vi "User Defined Errors.vi"(8 "error in (no error)":errorcluster, 9 "Parameter 2":string, 10 "Parameter 1":string, 11 "Error Code (0)":i32=-1) -> (0 "error out":errorcluster)   [LabVIEW 2024]
doc: "Returns the error by specifying the error code."
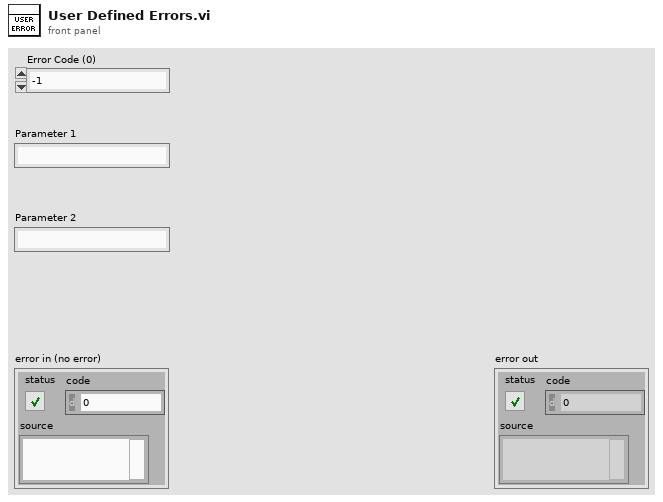
[diagram p1: front panel]
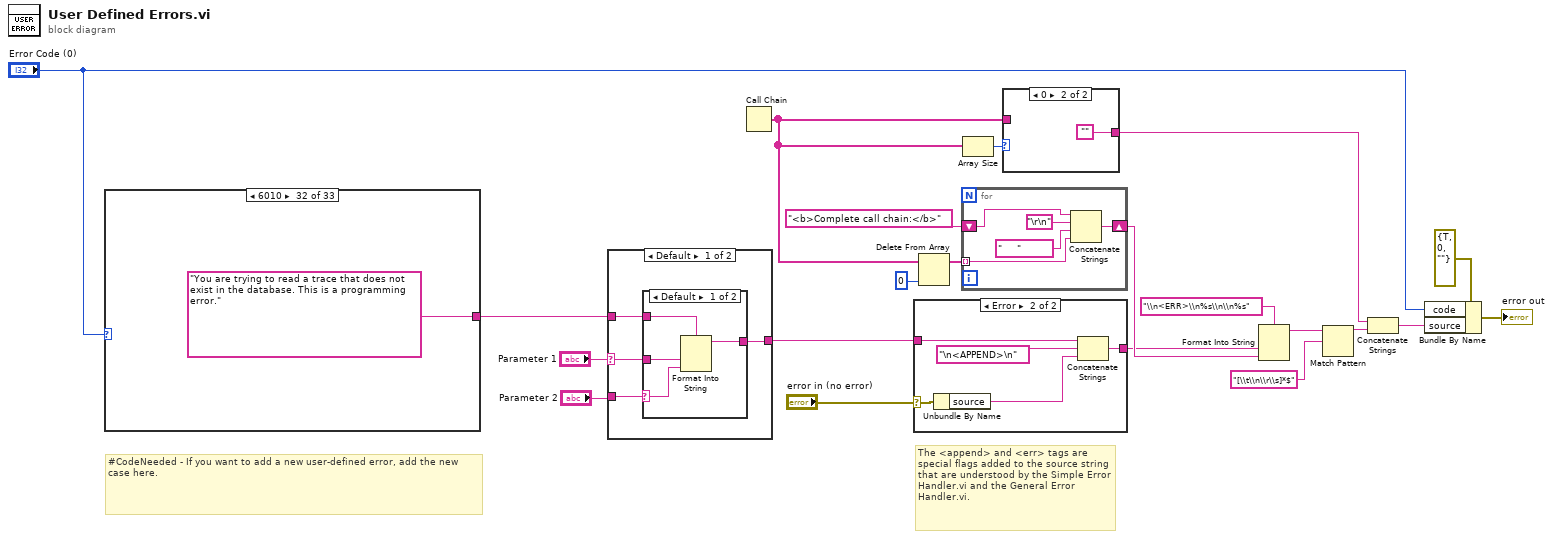
[diagram p0: block diagram]
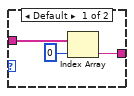
[diagram p2: hidden frame]
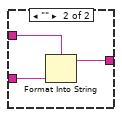
[diagram p4: hidden frame]
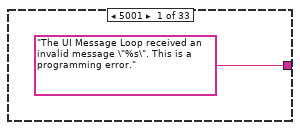
[diagram p6: hidden frame]
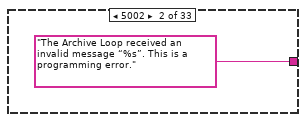
[diagram p7: hidden frame]
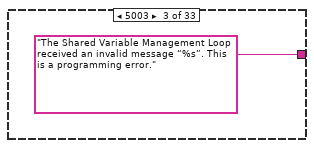
[diagram p8: hidden frame]
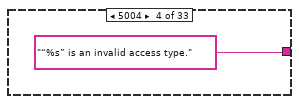
[diagram p9: hidden frame]
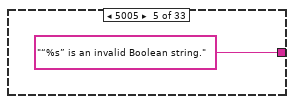
[diagram p10: hidden frame]
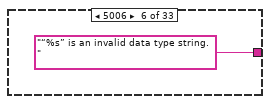
[diagram p11: hidden frame]
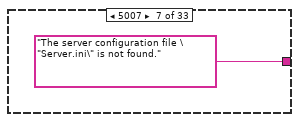
[diagram p12: hidden frame]
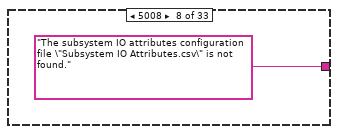
[diagram p13: hidden frame]
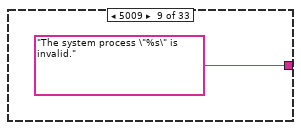
[diagram p14: hidden frame]
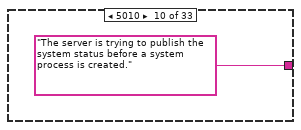
[diagram p15: hidden frame]
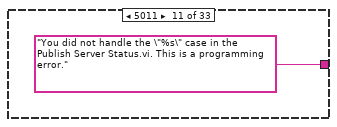
[diagram p16: hidden frame]
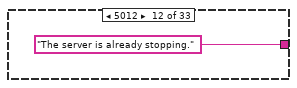
[diagram p17: hidden frame]
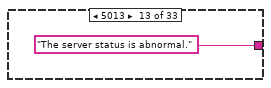
[diagram p18: hidden frame]
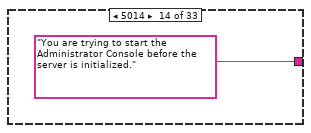
[diagram p19: hidden frame]
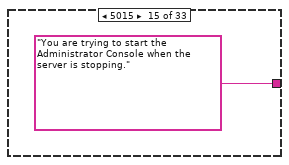
[diagram p20: hidden frame]
diagram:
  # "#CodeNeeded - If you want to add a new user-defined error, add the new case here."
  # "The <append> and <err> tags are special flags added to the source string that are understood by the Simple Error Handler.vi and the General Error Handler.vi."
  n1 = case shown="6010" "Error Code (0)" {
    selector: "Error Code (0)" -> [_ _ _ _ _ _ _ _ _ _ _ _ _ _ _ _ _ _ _ _ _ _ _ _ _ _ _ _ _ _ _ _ w55]
    tunnel: ["The UI Message Loop received an invalid message \"%s\". This is a programming error." ("Invalid Logging Message") "The Archive Loop received an invalid message “%s”. This is a programming error." ("Invalid Logging Message") "The Shared Variable Management Loop received an invalid message “%s”. This is a programming error." ("Unknown Message Error Text") "“%s” is an invalid access type." ("Invalid Logging Message") "“%s” is an invalid Boolean string." ("Invalid Logging Message") "“%s” is an invalid data type string. " ("Invalid Logging Message") "The server configuration file \"Server.ini\" is not found." ("Invalid Logging Message") "The subsystem IO attributes configuration file \"Subsystem IO Attributes.csv\" is not found." ("Invalid Logging Message") "The system process \"%s\" is invalid." ("Invalid Logging Message") "The server is trying to publish the system status before a system process is created." ("Invalid Logging Message") "You did not handle the \"%s\" case in the Publish Server Status.vi. This is a programming error." ("message") "The server is already stopping." ("message") "The server status is abnormal." ("error message (\"\")") "You are trying to start the Administrator Console before the server is initialized." ("message") "You are trying to start the Administrator Console when the server is stopping." ("message") "The shared variable management failed to initialize." ("Invalid Logging Message") "The system configuration update failed." ("Invalid Logging Message") "A timer error occurred." ("Invalid Logging Message") "The archival failed." ("message") "The Administrator Console received an invalid message \"%s\". This is a programming error." ("message") "The archival configuration update failed." ("message") "The archival initialization failed." ("message") "The Message Handling Loop in the Client Main.vi received an invalid message “%s”. This is a programming error." ("Invalid Logging Message") "The Message Handling Loop in the Detailed View.vi received an invalid message “%s”. This is a programming error." ("Invalid Logging Message") "You are trying to switch to another detailed subview  with the \"%s\" command. But you did not create a corresponding switching case in the Open Subview VI Reference.vi. This is a programming error." ("message") "The string \"%s\" already exists in the list." "The string \"%s\" is already removed from the list." "Failed to read the historical data." "The array size of the data exceeds the maximum value of the array size. This is a programming error." "The client configuration file \"Client.ini\" is not found." ("message") "You are trying to bind the control \"%s\" to an item. But you did not create a corresponding binding case in advance. This is a programming error." ("message") "You are trying to read a trace that does not exist in the database. This is a programming error." ("message") w54] -> w21
    frame 5001 {
    }
    frame 5002 {
    }
    frame 5003 {
    }
    frame 5004 {
    }
    frame 5005 {
    }
    frame 5006 {
    }
    frame 5007 {
    }
    frame 5008 {
    }
    frame 5009 {
    }
    frame 5010 {
    }
    frame 5011 {
    }
    frame 5012 {
    }
    frame 5013 {
    }
    frame 5014 {
    }
    frame 5015 {
    }
    frame 5016 {
    }
    frame 5017 {
    }
    frame 5018 {
    }
    frame 5019 {
    }
    frame 5020 {
    }
    frame 5021 {
    }
    frame 5022 {
    }
    frame 6001 {
    }
    frame 6002 {
    }
    frame 6003 {
    }
    frame 6004 {
    }
    frame 6005 {
    }
    frame 6006 {
    }
    frame 6007 {
    }
    frame 6008 {
    }
    frame 6009 {
    }
    frame 6010 {
    }
    frame Default {
      n2 = Format Into String(format string="The error code \"%d\" is not defined. " ("Unknown Message Error Text"), w55) -> (resulting string=w54:string)  [unwired: 2 in, 1 out]
    }
  }
  n3 = case shown="Default" "Parameter 1" {
    selector: "Parameter 1" -> [w58 _]
    tunnel: [w60 w68] -> w5
    tunnel: w21 -> [w59 w68]
    tunnel: "Parameter 2" -> [w57 _]
    frame Default {
      n4 = case shown="Default" w57 {
        selector: w57 -> [w61 _]
        tunnel: w58 -> [w64 w67]
        tunnel: [w63 w66] -> w60
        tunnel: w59 -> [w62 w65]
        frame Default {
          n5 = Format Into String(format string=w62, w64, w61) -> (resulting string=w63:string)  [unwired: 2 in, 1 out]
        }
        frame "" {
          n6 = Format Into String(format string=w65, w67) -> (resulting string=w66:string)  [unwired: 2 in, 1 out]
        }
      }
    }
    frame "" {
    }
  }
  n7 = Call Chain() -> (call chain=w2:string[])
  n8 = case shown="Error" "error in (no error)" {
    selector: "error in (no error)" -> [_ w73]
    tunnel: [w69 w74] -> w4
    tunnel: w5 -> [w69 w70]
    frame No Error {
    }
    frame Error {
      n9 = Unbundle By Name(w73) -> ("source"=w72:string)
      n10 = Concatenate Strings(w70, "\n<APPEND>\n", w72) -> (w74:string)
    }
  }
  n11 = Delete From Array(array=w2, index=0) -> (array with subset deleted=w13:string[])  [unwired: 1 in, 1 out]
  n12 = for {
    tunnel: w13 -> [w76] mode=indexing
    shift-right: [w79] -> w7
    shift-left: "<b>Complete call chain:</b>" ("call chain header") -> [w77]
    n13 = Concatenate Strings(w77, "\r\n", "     ", w76) -> (w79:string)
  }
  n14 = Array Size(array=w2) -> (size(s)=w3:i32)
  n15 = case shown="0" w3 {
    tunnel: w2 -> [w81 _]
    tunnel: [w80 ""] -> w1
    frame Default {
      n16 = Index Array(array=w81, index=0) -> (element=w80:string)
    }
    frame 0 {
    }
  }
  n17 = Format Into String(format string="\\n<ERR>\\n%s\\n\\n%s", w4, w7) -> (resulting string=w15:string)  [unwired: 2 in, 1 out]
  n18 = Match Pattern(string=w15, regular expression="[\\t\\n\\r\\s]*$") -> (before substring=w6:string)  [unwired: 1 in, 3 out]
  n19 = Concatenate Strings(w1, w6) -> (w9:string)
  n20 = Bundle By Name(cluster=errorcluster {"status"=TRUE, "code"=0, "source"=""} ("error constant"), "code"="Error Code (0)", "source"=w9) -> (→"error out":errorcluster)
